vi "FPGA_Main.vi"() -> ()   [LabVIEW 2018]
uses:
  <vilib>/Platform/TimedLoop/XDataNode/timing_clust.ctl
  <vilib>/Platform/TimedLoop/XDataNode/nitl_modes.ctl
  <vilib>/Platform/TimedLoop/XDataNode/wakeup.ctl
  <vilib>/rvi/Emulation/niFpgaGetClockAttributes.vi
  <vilib>/rvi/Emulation/niFpgaSctlEmulationGetInTimedLoop.vi
  <vilib>/rvi/Emulation/niFpgaEmulationReportErrorSimple.vi
  <vilib>/rvi/Emulation/niFpgaProcessEmulError.vi
  <vilib>/rvi/eio/common/nirviEmuTemplateMethod_errors.vi
  <vilib>/rvi/Emulation/niFpgaCriticalErrorInLSC.vi
  <vilib>/platform/TimedLoop/XDataNode/XDataNode.xnode
  <vilib>/eio/EIONode/EIONode.xnode
  <vilib>/Platform/TimedLoop/XDataNode/XDNodeRunTimeDep.lvlib
panel:
  out "speed":i16
  in  "dt_pwm_us":u32=200 caption="Count(uSec)"
  out "busy":bool
  in  "dt_m_us":u32=100 caption="dt_M_us"
  in  "setpoint":i16
  in  "dead band":i16=3
  in  "inv":bool=TRUE
  out "AI0":u16
  out "dai":i16
  out "backward":bool
  out "pos":i16=1867
  out "err cnt":i16=13
  in  "reset":bool
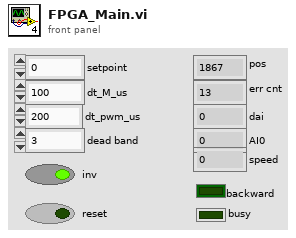
[diagram p1: front panel]
types:
  T1 = typedef "XDNodeRunTimeDep.lvlib/timing_clust.ctl" = cluster{"Expected End [f-1]":u64, "Actual End [f-1]":u64, "Finished Late? [f-1]":bool, "Expected End [i-1]":u64, "Actual End [i-1]":u64, "Finished Late? [i-1]":bool, "Expected Start [i]":u64, "Actual Start [i]":u64, "Expected Start [f]":u64, "Actual Start [f]":u64, "Source Name":string, "Structure Name":string, "Period":i64, "Deadline":i64, "Offset":i64, "Start":i64, "Priority":i32, "Timeout":i32, "Mode":T2, "Wakeup Reason":T3, "Error":errorcluster, "Source Type":string, "Secondary Source Type":string, "Global End Time":u64, "Global Start Time":u64, "Frame Duration":u64, "Iteration Duration":u64, "Assigned CPU":i32, "I/O Scan Engine Mode":u32}
  T2 = typedef "XDNodeRunTimeDep.lvlib/nitl_modes.ctl" = enum32{"No Change", "Process missed periods, maintain original phase", "Discard missed periods, maintain original phase", "Process missed periods, ignore original phase", "Discard missed periods, ignore original phase"}
  T3 = typedef "XDNodeRunTimeDep.lvlib/wakeup.ctl" = enum32{"Normal", "Aborted", "Asynchronous wakeup", "Timing source error", "Timed loop error", "Timeout"}
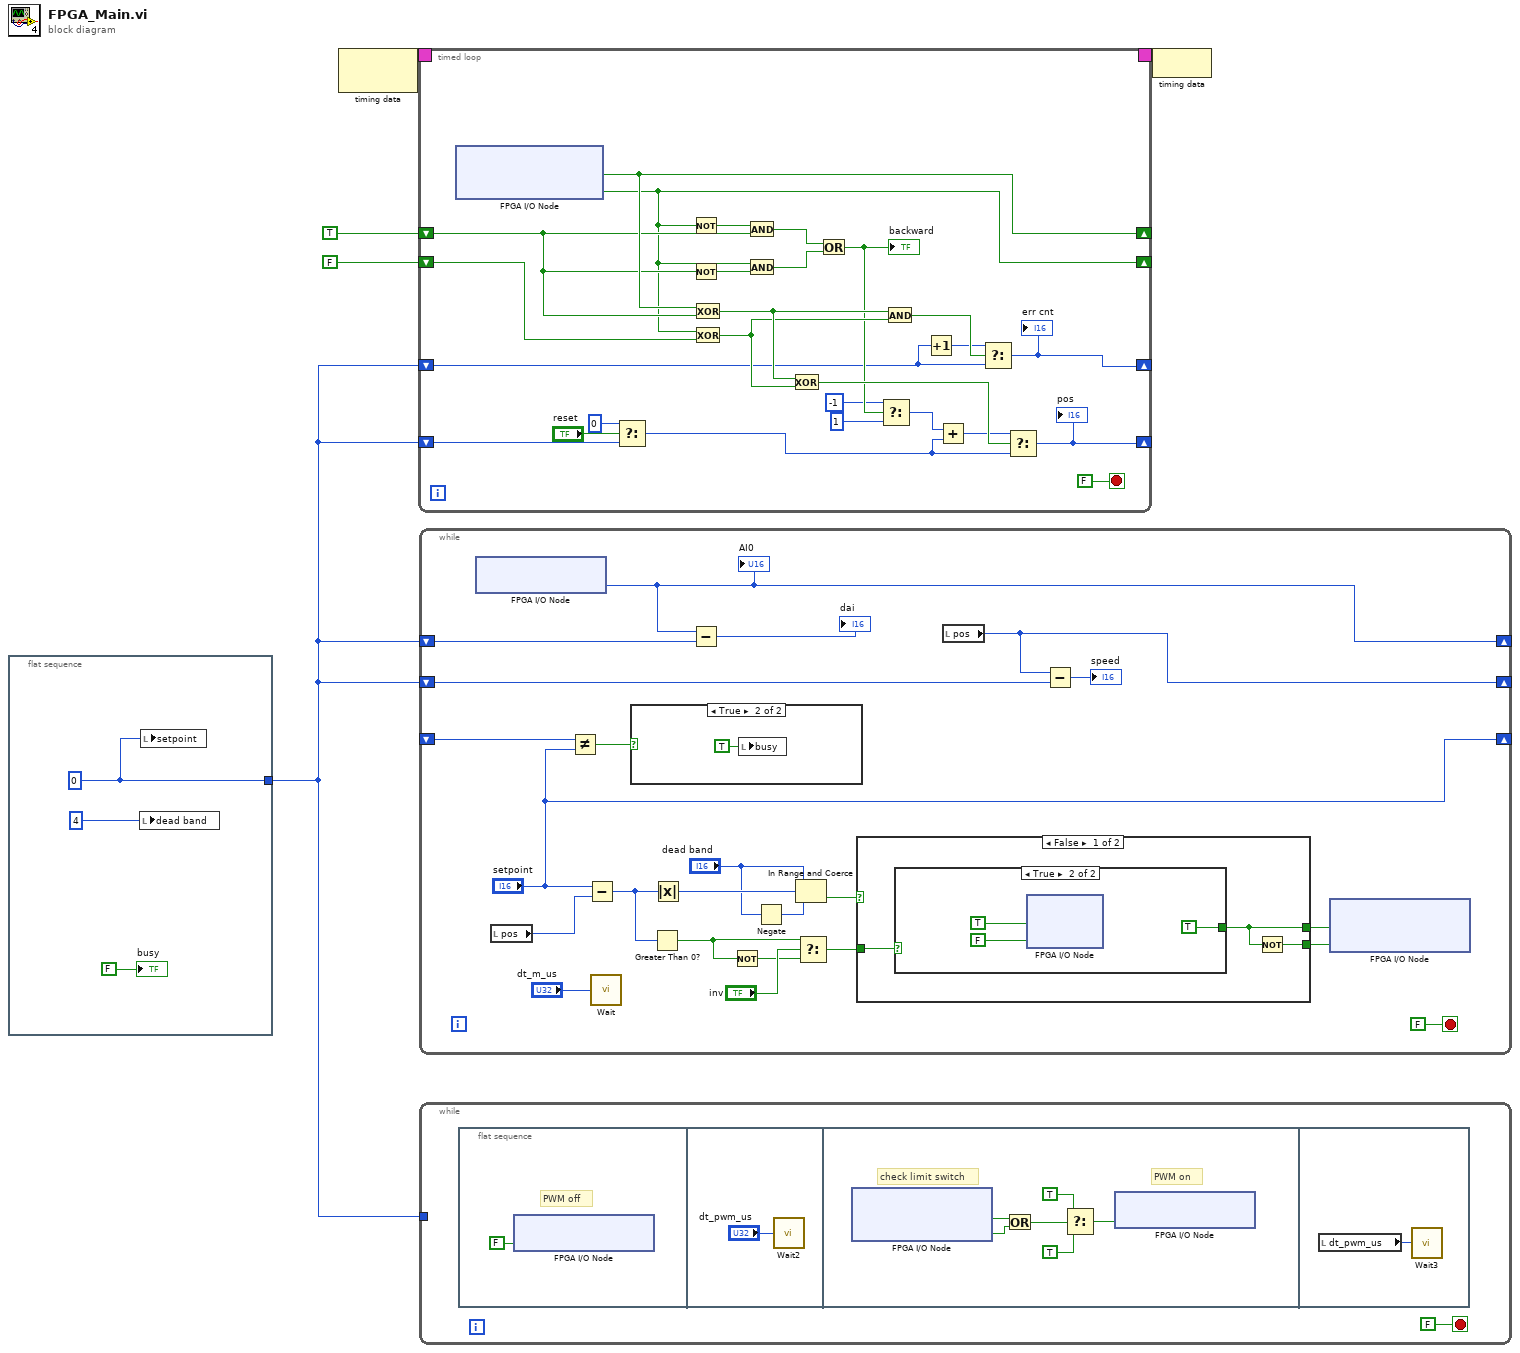
[diagram p0: block diagram]
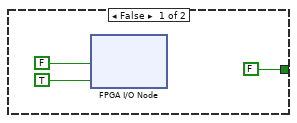
[diagram p3: hidden frame]
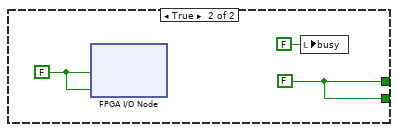
[diagram p4: hidden frame]
diagram:
  n1 = flat-sequence {
    tunnel: [w7] -> w1
    frame #0 {
      w7 = i16 0
      n2 = local write "dead band"(i16 4 ("dead band")) -> ()
      n3 = local write "setpoint"(w7) -> ()
      "busy" <- FALSE ("status")
    }
  }
  n4 = node-c288() -> (w5:T1)  [unwired: 1 in]
  n5 = timed-loop {
    timing: w5 -> [_]
    timing-out: [_] -> w4
    shift-right: [w29] -> _
    shift-left: TRUE ("ConnectorA/DIO11") -> [w28]
    shift-right: [w27] -> _
    shift-left: FALSE ("ConnectorA/DIO12") -> [w26]
    shift-right: [w22] -> _
    shift-left: w1 -> [w11]
    shift-right: [w13] -> _
    shift-left: w1 -> [w14]
    stop <- FALSE stop-if-true
    n6 = xnode "FPGA I/O Node"() -> ("ConnectorA/DIO11"=w29:bool, "ConnectorA/DIO12"=w27:bool)  [unwired: 2 in, 2 out]
    n7 = Select(t=i16 0, s="reset", f=w11) -> (s? t:f=w9:i16)
    n8 = Not(x=w27) -> (.not. x?=w33:bool)
    n9 = Not(x=w28) -> (.not. x?=w32:bool)
    n10 = Exclusive Or(1:w28, 2:w29) -> (0:w25:bool)
    n11 = Exclusive Or(1:w26, 2:w27) -> (0:w24:bool)
    n12 = And(x=w33, y=w28) -> (x .and. y?=w30:bool)
    n13 = And(x=w27, y=w32) -> (x .and. y?=w31:bool)
    n14 = Exclusive Or(1:w24, 2:w25) -> (0:w23:bool)
    n15 = Or(x=w30, y=w31) -> (x .or. y?=w21:bool)
    "backward" <- w21
    n16 = Select(t=i16 -1, s=w21, f=i16 1) -> (s? t:f=w18:i16)
    n17 = And(x=w25, y=w24) -> (x .and. y?=w16:bool)
    n18 = Increment(x=w14) -> (x+1=w15:i16)
    n19 = Add(x=w18, y=w9) -> (x+y=w17:i16)
    n20 = Select(t=w15, s=w16, f=w14) -> (s? t:f=w13:i16)
    "err cnt" <- w13
    n21 = Select(t=w17, s=w23, f=w9) -> (s? t:f=w22:i16)
    "pos" <- w22
  }
  n22 = while {
    shift-right: ["setpoint"] -> _
    shift-left: _ -> [w44]
    shift-right: [w42] -> _
    shift-left: w1 -> [w41]
    shift-right: [w39] -> _
    shift-left: w1 -> [w38]
    stop <- FALSE stop-if-true
    n23 = xnode "FPGA I/O Node"() -> ("ConnectorA/AI0"=w42:u16)  [unwired: 1 in, 1 out]
    "AI0" <- w42
    n24 = local read "pos"() -> (w55:i16)
    n25 = Not Equal?(x=w44, y="setpoint") -> (x != y?=w43:bool)
    n26 = Subtract(x="setpoint", y=w55) -> (x-y=w46:i16)
    n27 = call "Wait"("Count(uSec)"="dt_m_us") -> ()  [unwired: 1 out]
    n28 = case shown="True" w43 {
      frame False {
      }
      frame True {
        n29 = local write "busy"(TRUE ("busy")) -> ()
      }
    }
    n30 = Greater Than 0?(x=w46) -> (x > 0?=w48:bool)
    n31 = Absolute Value(x=w46) -> (abs(x)=w54:i16)
    n32 = Subtract(x=w42, y=w41) -> (x-y=→"dai":u16)
    n33 = Not(x=w48) -> (.not. x?=w49:bool)
    n34 = Negate(x="dead band") -> (-x=w53:i16)
    n35 = In Range and Coerce(upper limit="dead band", x=w54, lower limit=w53) -> (In Range?=w51:bool)  [unwired: 1 out]
    n36 = Select(t=w48, s="inv", f=w49) -> (s? t:f=w47:bool)
    n37 = case shown="False" w51 {
      tunnel: [w63 w72] -> w57
      tunnel: [w62 w72] -> w56
      tunnel: w47 -> [w61 _]
      frame False {
        n38 = case shown="True" w61 {
          tunnel: [FALSE ("dir") TRUE ("dir")] -> w62
          frame False {
            n39 = xnode "FPGA I/O Node"("LED0"=FALSE, "LED1"=TRUE) -> ()  [unwired: 2 in, 2 out]
          }
          frame True {
            n40 = xnode "FPGA I/O Node"("LED0"=TRUE, "LED1"=FALSE) -> ()  [unwired: 2 in, 2 out]
          }
        }
        n41 = Not(x=w62) -> (.not. x?=w63:bool)
      }
      frame True {
        w70 = FALSE ("LED0")
        w72 = FALSE ("dir")
        n42 = xnode "FPGA I/O Node"("LED0"=w70, "LED1"=w70) -> ()  [unwired: 2 in, 2 out]
        n43 = local write "busy"(FALSE ("busy")) -> ()
      }
    }
    n44 = local read "pos"() -> (w39:i16)
    n45 = Subtract(x=w39, y=w38) -> (x-y=→"speed":i16)
    n46 = xnode "FPGA I/O Node"("ConnectorA/DIO6"=w56, "ConnectorA/DIO5"=w57) -> ()  [unwired: 2 in, 2 out]
  }
  n47 = while {
    tunnel: w1 -> [_]
    stop <- FALSE stop-if-true
    n48 = flat-sequence {
      frame #0 {
        # "PWM off"
        n49 = xnode "FPGA I/O Node"("ConnectorA/DIO8"=FALSE) -> ()  [unwired: 1 in, 1 out]
      }
      frame #1 {
        n50 = call "Wait2"("Count(uSec)"="dt_pwm_us") -> ()  [unwired: 1 out]
      }
      frame #2 {
        # "check limit switch"
        # "PWM on"
        n51 = xnode "FPGA I/O Node"() -> ("ConnectorA/DIO0"=w80:bool, "ConnectorA/DIO1"=w81:bool)  [unwired: 2 in, 2 out]
        n52 = Or(x=w80, y=w81) -> (x .or. y?=w79:bool)
        n53 = Select(t=TRUE, s=w79, f=TRUE ("ConnectorA/DIO8")) -> (s? t:f=w77:bool)
        n54 = xnode "FPGA I/O Node"("ConnectorA/DIO8"=w77) -> ()  [unwired: 1 in, 1 out]
      }
      frame #3 {
        n55 = local read "dt_pwm_us"() -> (w82:u32)
        n56 = call "Wait3"("Count(uSec)"=w82) -> ()  [unwired: 1 out]
      }
    }
  }
  n57 = node-c288(w4) -> ()
